vi "test-simpleSpreadsheet.vi"() -> ()   [LabVIEW 2009]
uses:
  <vilib>/Utility/sysdir.llb/System Directory Type.ctl
  ooCalc/ooCalc.lvclass
panel:
  in  "position 2":cluster{"Row":u32, "Column":u32}
  in  "position":cluster{"Row":u32, "Column":u32}
  in  "Sheet Name":string="sheet1"
  in  "text":string="report"
  out "Calc error":errorcluster
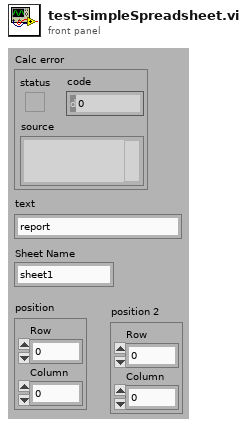
[diagram p1: front panel]
types:
  T1 = typedef "System Directory Type.ctl" = i32
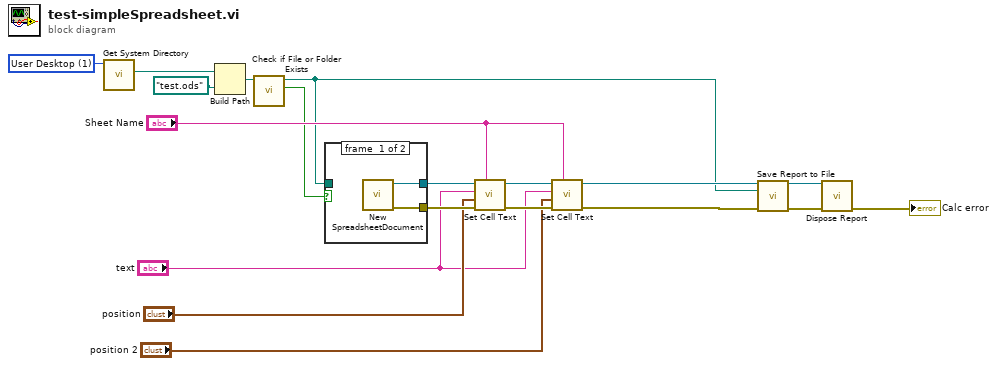
[diagram p0: block diagram]
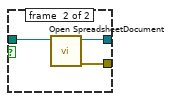
[diagram p2: hidden frame]
diagram:
  w19 = T1 1 items=["User Home", "User Desktop", "User Documents", "User Application Data", "User Preferences", "User Temporary", "Public Documents", "Public Application Data", "Public Preferences", "System Core Libraries", "System Installed Libraries", "Application Files", "Boot Volume Root"] ("system directory type")
  n1 = call <vilib>:"Get System Directory.vi"("system directory type"=w19) -> ("system directory"=w18:path)  [unwired: 10 in]
  n2 = Build Path(base path=w18, name or relative path=path "test.ods") -> (appended path=w3:path)
  n3 = call <vilib>:"Check if File or Folder Exists.vi"("path"=w3) -> ("file or folder exists?"=w2:bool, "dup path"=w1:path)  [unwired: 8 in, 1 out]
  n4 = case shown="True" w2 {
    tunnel: [w21 w24] -> w16
    tunnel: [w20 w22] -> w15
    tunnel: w1 -> [_ w23]
    frame #0 {
      n5 = call "New SpreadsheetDocument.vi"() -> ("error out"=w20:errorcluster, "ooCalc out"=w21:refnum<class "ooCalc.lvclass">)  [unwired: 10 in]
    }
    frame #1 {
      n6 = call "Open SpreadsheetDocument.vi"("filepath"=w23) -> ("error out"=w22:errorcluster, "ooCalc out"=w24:refnum<class "ooCalc.lvclass">)  [unwired: 9 in]
    }
  }
  n7 = call-dynamic "Set Cell Text.vi"("Sheet Name"="Sheet Name", "error in (no error)"=w15, "position"="position", "text"="text", "report in"=w16) -> ("error out"=w12:errorcluster, "report out"=w13:refnum<class "ooCalc.lvclass">)  [unwired: 5 in]
  n8 = call-dynamic "Set Cell Text.vi"("Sheet Name"="Sheet Name", "error in (no error)"=w12, "position"="position 2", "text"="text", "report in"=w13) -> ("error out"=w8:errorcluster, "report out"=w7:refnum<class "ooCalc.lvclass">)  [unwired: 5 in]
  n9 = call-dynamic "Save Report to File.vi"("report in"=w7, "report file path"=w1, "error in (no error)"=w8) -> ("report out"=w6:refnum<class "ooCalc.lvclass">, "error out"=w5:errorcluster)  [unwired: 11 in]
  n10 = call-dynamic "Dispose Report.vi"("report in"=w6, "error in (no error)"=w5) -> ("error out"=→"Calc error":errorcluster)  [unwired: 13 in]
